vi "均值角点排序.vi"() -> ()   [LabVIEW 2014]
panel:
  in  "均值角点":cluster{"X":sgl, "Y":sgl}[](array[cluster])
  out "数组":cluster{"X":sgl, "Y":sgl}[][](array[cluster])
  in  "有序均值角点":cluster{"X":sgl, "Y":sgl}[](array[cluster])=[{"X"=26.153654, "Y"=19.799763}, {"X"=117.94913, "Y"=18.043228}, {"X"=210.42528, "Y"=16.104532}, {"X"=303.14487, "Y"=16.804981}, {"X"=395.8317, "Y"=14.265327}, {"X"=488.088, "Y"=12.905719}, {"X"=581.6167, "Y"=12.267984}, {"X"=674.5895, "Y"=12.91218}, {"X"=767.76306, "Y"=10.226602}, {"X"=860.28406, "Y"=8.9823675}, {"X"=952.73627, "Y"=9.615947}, {"X"=1046.6309, "Y"=7.880585}, {"X"=1138.7231, "Y"=8.074149}, {"X"=1231.7189, "Y"=7.871906}, {"X"=1322.7467, "Y"=6.319392}, {"X"=1415.9888, "Y"=7.2800922}, {"X"=1510.8711, "Y"=11.122694}, {"X"=26.5582, "Y"=112.33133}, {"X"=117.30896, "Y"=113.06552}, {"X"=210.60878, "Y"=109.2212}, {"X"=303.7148, "Y"=108.67336}, {"X"=397.0007, "Y"=106.83352}, {"X"=488.98993, "Y"=105.69125}, {"X"=582.4377, "Y"=105.0102}, {"X"=675.4467, "Y"=103.79006}, {"X"=768.209, "Y"=102.46854}, {"X"=861.8379, "Y"=102.300735}, {"X"=954.83936, "Y"=101.902596}, {"X"=1047.6487, "Y"=100.940865}, {"X"=1140.4517, "Y"=100.67957}, {"X"=1233.0221, "Y"=100.59138}, {"X"=1324.6829, "Y"=99.951775}, {"X"=1417.1527, "Y"=99.93431}, {"X"=1508.0281, "Y"=99.89758}, {"X"=27.254702, "Y"=204.95152}, {"X"=119.1949, "Y"=204.1937}, {"X"=211.73006, "Y"=200.71664}, {"X"=305.2511, "Y"=200.301}, {"X"=397.0177, "Y"=199.83902}, {"X"=490.28326, "Y"=197.84201}, {"X"=583.30597, "Y"=197.79129}, {"X"=676.3955, "Y"=198.59354}, {"X"=769.5109, "Y"=196.1777}, {"X"=862.86005, "Y"=195.38493}, {"X"=955.83563, "Y"=193.68704}, {"X"=1048.5593, "Y"=193.363}, {"X"=1141.3936, "Y"=195.22557}, {"X"=1233.9485, "Y"=194.60788}, {"X"=1326.1038, "Y"=192.30125}, {"X"=1418.2493, "Y"=192.26222}, {"X"=1509.9326, "Y"=193.04053}, {"X"=27.658695, "Y"=297.54025}, {"X"=120.20574, "Y"=296.1477}, {"X"=212.2937, "Y"=296.94568}, {"X"=305.33676, "Y"=294.0102}, {"X"=397.98285, "Y"=292.05518}, {"X"=489.92435, "Y"=292.0649}, {"X"=584.1639, "Y"=290.7395}, {"X"=677.1442, "Y"=290.02478}, {"X"=770.44354, "Y"=288.9485}, {"X"=863.7642, "Y"=288.35236}, {"X"=956.54846, "Y"=288.5216}, {"X"=1049.5681, "Y"=286.9658}, {"X"=1142.373, "Y"=286.12158}, {"X"=1235.4694, "Y"=284.9839}, {"X"=1327.159, "Y"=284.9216}, {"X"=1419.3372, "Y"=284.41812}, {"X"=1510.9773, "Y"=284.24063}, {"X"=27.92012, "Y"=390.14224}, {"X"=122.703026, "Y"=387.3263}, {"X"=212.80882, "Y"=390.21768}, {"X"=306.16815, "Y"=385.03027}, {"X"=398.8617, "Y"=387.05548}, {"X"=491.99292, "Y"=384.90576}, {"X"=585.08325, "Y"=383.7588}, {"X"=677.5269, "Y"=383.44208}, {"X"=771.5025, "Y"=382.54758}, {"X"=864.2984, "Y"=381.2901}, {"X"=957.39575, "Y"=379.49994}, {"X"=1050.6702, "Y"=380.41113}, {"X"=1143.0787, "Y"=377.24036}, {"X"=1235.6982, "Y"=379.10297}, {"X"=1328.1119, "Y"=377.8064}, {"X"=1420.1188, "Y"=377.09894}, {"X"=1512.4355, "Y"=375.9555}, {"X"=29.905834, "Y"=484.79666}, {"X"=122.00639, "Y"=482.18176}, {"X"=214.56398, "Y"=480.8908}, {"X"=307.15845, "Y"=479.90918}, {"X"=400.02325, "Y"=478.98444}, {"X"=493.61395, "Y"=478.45593}, {"X"=585.83746, "Y"=476.98575}, {"X"=678.4713, "Y"=478.21262}, {"X"=771.99445, "Y"=475.16855}, {"X"=865.5039, "Y"=474.58887}, {"X"=958.48724, "Y"=473.41083}, {"X"=1050.7454, "Y"=472.20322}, {"X"=1144.2859, "Y"=472.09476}, {"X"=1236.1927, "Y"=470.99536}, {"X"=1328.5546, "Y"=471.20746}, {"X"=1419.2249, "Y"=469.91147}, {"X"=1513.1338, "Y"=469.6233}, {"X"=31.062618, "Y"=575.79315}, {"X"=121.209305, "Y"=574.8945}, {"X"=215.5965, "Y"=573.68176}, {"X"=308.0694, "Y"=572.8096}, {"X"=397.7425, "Y"=572.5649}, {"X"=494.02304, "Y"=571.0017}, {"X"=588.4636, "Y"=570.0561}, {"X"=680.02856, "Y"=569.1081}, {"X"=771.7187, "Y"=568.1693}, {"X"=865.6112, "Y"=567.38727}, {"X"=959.4974, "Y"=566.2953}, {"X"=1051.9573, "Y"=565.8523}, {"X"=1144.1035, "Y"=563.87573}, {"X"=1237.4873, "Y"=564.21716}, {"X"=1329.2723, "Y"=563.413}, {"X"=1421.7517, "Y"=562.54346}, {"X"=1513.3787, "Y"=561.71606}, {"X"=31.646376, "Y"=668.3817}, {"X"=124.28865, "Y"=667.6554}, {"X"=216.63431, "Y"=666.56476}, {"X"=309.2264, "Y"=665.89246}, {"X"=402.76028, "Y"=664.39764}, {"X"=494.94122, "Y"=664.08325}, {"X"=588.0022, "Y"=663.2181}, {"X"=681.0126, "Y"=662.0835}, {"X"=773.83704, "Y"=662.2445}, {"X"=868.4772, "Y"=660.12537}, {"X"=959.81104, "Y"=660.26514}, {"X"=1052.9458, "Y"=657.36487}, {"X"=1145.1924, "Y"=657.4666}, {"X"=1237.9401, "Y"=656.9574}, {"X"=1330.3198, "Y"=656.0417}, {"X"=1422.6621, "Y"=654.47705}, {"X"=1513.1232, "Y"=654.56964}, {"X"=33.171947, "Y"=760.686}, {"X"=125.15056, "Y"=760.2781}, {"X"=217.85513, "Y"=759.4324}, {"X"=310.3773, "Y"=758.6699}, {"X"=404.78345, "Y"=757.8375}, {"X"=496.18146, "Y"=756.2565}, {"X"=588.31995, "Y"=756.5905}, {"X"=681.62964, "Y"=754.6544}, {"X"=774.24097, "Y"=754.68195}, {"X"=867.75037, "Y"=753.7057}, {"X"=960.8959, "Y"=751.4333}, {"X"=1053.5225, "Y"=753.06836}, {"X"=1146.2054, "Y"=750.27655}, {"X"=1236.9874, "Y"=749.2309}, {"X"=1332.7157, "Y"=748.58545}, {"X"=1422.7683, "Y"=748.6518}, {"X"=1514.5779, "Y"=746.4824}, {"X"=33.17179, "Y"=852.7198}, {"X"=127.01915, "Y"=852.697}, {"X"=218.50732, "Y"=852.6804}, {"X"=311.56122, "Y"=852.0961}, {"X"=404.15656, "Y"=850.4625}, {"X"=496.9585, "Y"=849.85114}, {"X"=589.79974, "Y"=848.7624}, {"X"=683.08545, "Y"=847.43884}, {"X"=774.67126, "Y"=845.407}, {"X"=867.78253, "Y"=844.6072}, {"X"=962.5796, "Y"=845.97}, {"X"=1053.9875, "Y"=844.0548}, {"X"=1094.8916, "Y"=879.7679}, {"X"=1146.439, "Y"=843.13007}, {"X"=1239.023, "Y"=842.04205}, {"X"=1331.4849, "Y"=842.68604}, {"X"=1421.2545, "Y"=840.07336}, {"X"=1514.9934, "Y"=838.0892}, {"X"=35.592834, "Y"=945.0288}, {"X"=128.19093, "Y"=943.3827}, {"X"=221.42564, "Y"=944.74854}, {"X"=312.76135, "Y"=944.18274}, {"X"=405.28595, "Y"=942.8694}, {"X"=498.16595, "Y"=941.7714}, {"X"=590.5177, "Y"=941.55884}, {"X"=683.7365, "Y"=940.2383}, {"X"=776.82117, "Y"=939.21606}, {"X"=869.2016, "Y"=937.0309}, {"X"=962.3721, "Y"=937.5852}, {"X"=1054.0448, "Y"=936.20215}, {"X"=1147.3387, "Y"=935.5681}, {"X"=1239.2339, "Y"=934.34393}, {"X"=1328.8728, "Y"=928.75336}, {"X"=1423.3219, "Y"=932.1168}, {"X"=1514.9169, "Y"=930.89435}, {"X"=38.42954, "Y"=1037.6108}, {"X"=130.0787, "Y"=1037.184}, {"X"=221.89706, "Y"=1035.9017}, {"X"=314.19727, "Y"=1035.4048}, {"X"=406.37912, "Y"=1034.8766}, {"X"=499.1427, "Y"=1034.0789}, {"X"=592.01544, "Y"=1033.7883}, {"X"=683.73517, "Y"=1032.6879}, {"X"=777.4314, "Y"=1031.9902}, {"X"=870.0566, "Y"=1030.9749}, {"X"=962.8419, "Y"=1029.7119}, {"X"=1055.3657, "Y"=1028.0264}, {"X"=1147.8184, "Y"=1027.0546}, {"X"=1239.6836, "Y"=1025.8411}, {"X"=1331.8369, "Y"=1025.2474}, {"X"=1422.9252, "Y"=1024.1187}, {"X"=1514.7249, "Y"=1022.5082}, {"X"=39.908962, "Y"=1129.3448}, {"X"=132.16687, "Y"=1128.3557}, {"X"=223.63893, "Y"=1127.9443}, {"X"=315.1446, "Y"=1097.189}, {"X"=315.62305, "Y"=1128.1501}, {"X"=408.14102, "Y"=1129.0172}, {"X"=500.41644, "Y"=1126.0503}, {"X"=593.0427, "Y"=1125.741}, {"X"=685.8043, "Y"=1126.8809}, {"X"=778.4424, "Y"=1124.1752}, {"X"=869.13324, "Y"=1124.7325}, {"X"=963.6898, "Y"=1122.8662}, {"X"=1055.9153, "Y"=1119.2623}, {"X"=1148.0303, "Y"=1119.8373}, {"X"=1240.1152, "Y"=1118.4204}, {"X"=1332.13, "Y"=1115.1473}, {"X"=1423.6239, "Y"=1115.8408}, {"X"=1515.6151, "Y"=1115.1183}]
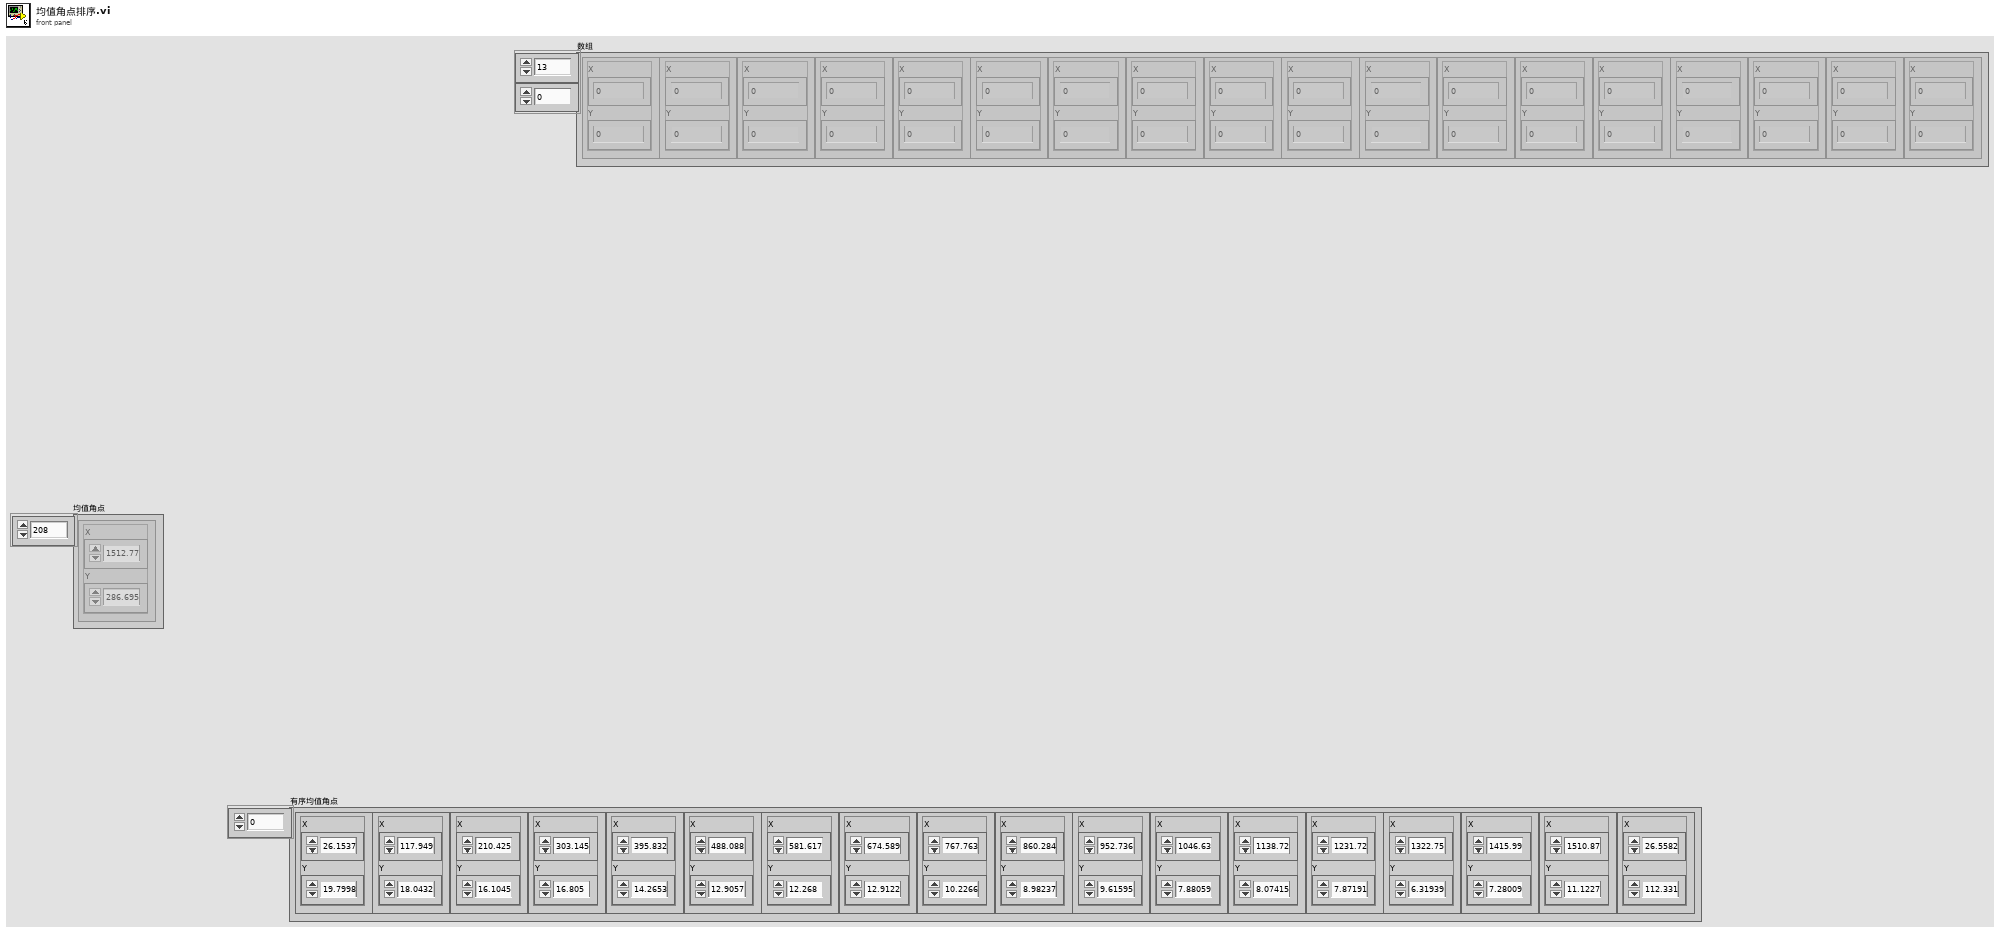
[diagram p1: front panel]
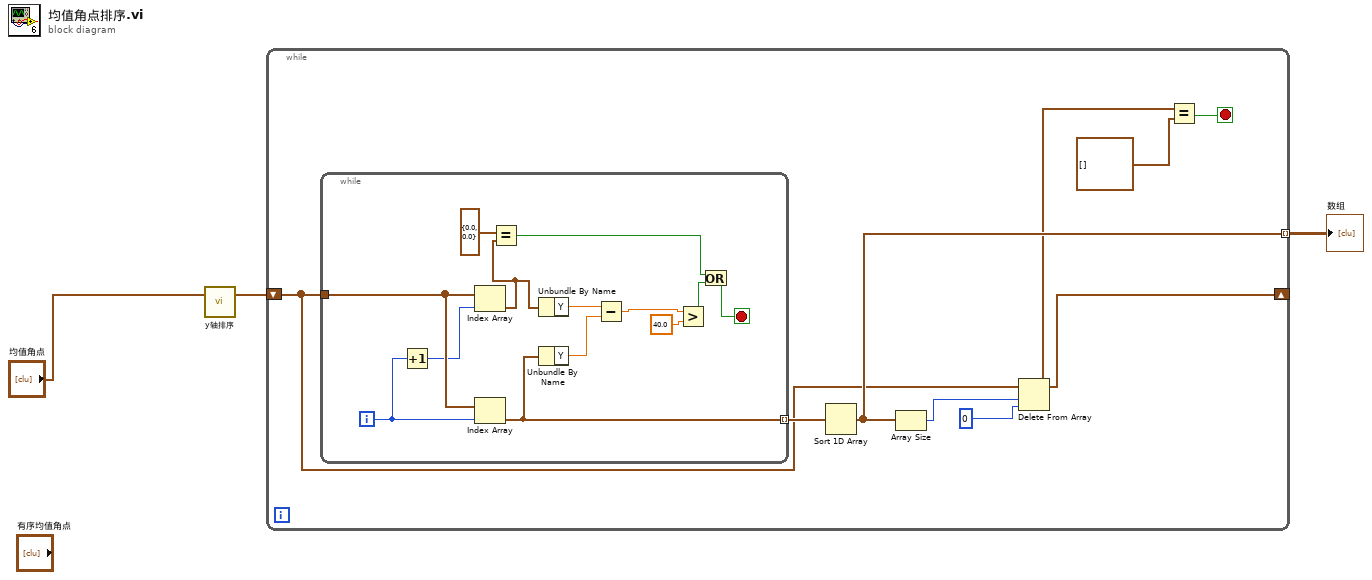
[diagram p0: block diagram]
diagram:
  n1 = call "y轴排序.vi"("均值角点"="均值角点") -> ("数组 2"=w2:cluster{"X":sgl, "Y":sgl}[])  [unwired: 2 in]
  n2 = while {
    shift-right: [w5] -> _
    shift-left: w2 -> [w4]
    tunnel: [w8] -> w3 mode=indexing
    stop <- w6 stop-if-true
    n3 = while {
      tunnel: w4 -> [w23]
      tunnel: [w19] -> w11 mode=indexing
      i -> [w24]
      stop <- w15 stop-if-true
      n4 = Increment(x=w24) -> (x+1=w22:i32)
      n5 = Index Array(array=w23, index=w22) -> (element=w14:cluster{"X":sgl, "Y":sgl})
      n6 = Index Array(array=w23, index=w24) -> (element=w19:cluster{"X":sgl, "Y":sgl})
      n7 = Equal?(x=cluster{"X":sgl, "Y":sgl} {"X"=0.0, "Y"=0.0}, y=w14) -> (x = y?=w12:bool)
      n8 = Unbundle By Name(w14) -> ("Y"=w17:sgl)
      n9 = Unbundle By Name(w19) -> ("Y"=w21:sgl)
      n10 = Subtract(x=w17, y=w21) -> (x-y=w18:sgl)
      n11 = Greater?(x=w18, y=sgl 40.0) -> (0:w16:bool)
      n12 = Or(x=w12, y=w16) -> (x .or. y?=w15:bool)
    }
    n13 = Sort 1D Array(array=w11) -> (sorted array=w8:cluster{"X":sgl, "Y":sgl}[])
    n14 = Array Size(array=w8) -> (size(s)=w10:i32)
    n15 = Delete From Array(array=w4, length=w10, index=0 ("索引")) -> (array with subset deleted=w5:cluster{"X":sgl, "Y":sgl}[])  [unwired: 1 out]
    n16 = Equal?(x=w5, y=cluster{"X":sgl, "Y":sgl}[] []) -> (x = y?=w6:bool)
  }
  "数组" <- w3
